vi "SubVI_Stepper_SMC100.vi"(0 "Function":enum16{"Initialize", "Position", "Close"}(ring), 1 "Offset QWP":dbl, 2 "New target position (units)":dbl format="%.2f", 3 "error in (no error)":errorcluster, 4 "Nom de ressource VISA":refnum<visa-resource-name>) -> (5 "Position":dbl, 6 "error out":errorcluster)   [LabVIEW 2025]
panel:
  in  "Timeout (ms)":u32=300
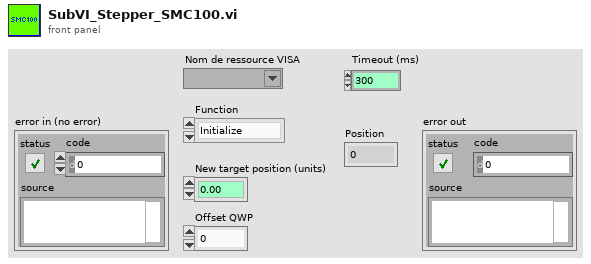
[diagram p1: front panel]
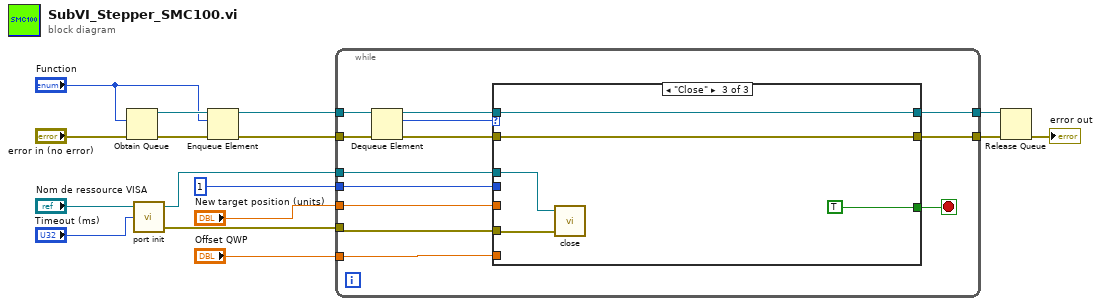
[diagram p0: block diagram]
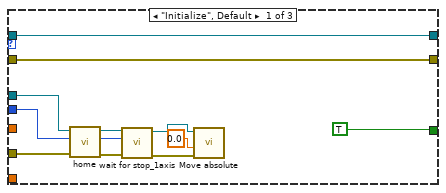
[diagram p2: hidden frame]
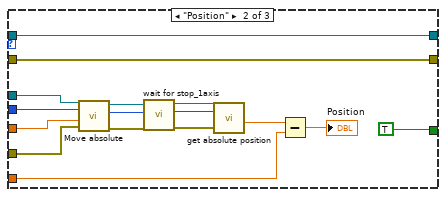
[diagram p3: hidden frame]
diagram:
  n1 = Obtain Queue(element data type="Function", error in (no error)="error in (no error)") -> (queue out=w15:refnum<queue>, error out=w16:errorcluster)  [unwired: 3 in, 1 out]
  n2 = call "port init.vi"("Timeout (ms)"="Timeout (ms)", "Nom de ressource VISA"="Nom de ressource VISA") -> ("error out"=w2:errorcluster, "Visa Handle"=w3:refnum<visa-resource-name>)  [unwired: 2 in]
  n3 = Enqueue Element(queue=w15, element="Function", error in (no error)=w16) -> (queue out=w13:refnum<queue>, error out=w12:errorcluster)  [unwired: 1 in, 1 out]
  n4 = while {
    tunnel: w13 -> [w29]
    tunnel: w12 -> [w28]
    tunnel: [w25] -> w11
    tunnel: [w23] -> w10
    tunnel: w3 -> [w21]
    tunnel: w2 -> [w20]
    tunnel: 1 ("Axis in") -> [w19]
    tunnel: "New target position (units)" -> [w18]
    tunnel: "Offset QWP" -> [w17]
    stop <- w22 stop-if-true
    n5 = Dequeue Element(queue=w29, error in (no error)=w28) -> (queue out=w24:refnum<queue>, element=w27:enum16{"Initialize", "Position", "Close"}, error out=w26:errorcluster)  [unwired: 1 in, 1 out]
    n6 = case shown="\"Close\"" w27 {
      tunnel: w26 -> [w40 w57 w61]
      tunnel: [w40 w57 w61] -> w25
      tunnel: w24 -> [w41 w56 w62]
      tunnel: [w41 w56 w62] -> w23
      tunnel: [TRUE TRUE TRUE] -> w22
      tunnel: w21 -> [w38 w46 w59]
      tunnel: w20 -> [w37 w44 w58]
      tunnel: w19 -> [w36 w45 _]
      tunnel: w18 -> [_ w43 _]
      tunnel: w17 -> [_ w42 _]
      frame "Initialize", Default {
        n7 = call <vilib>:"home.vi"("error in"=w37, "Axis in"=w36, "VISA Handle in"=w38) -> ("error out"=w33:errorcluster, "Axis out"=w34:i32, "VISA Handle out"=w35:refnum<visa-resource-name>)  [unwired: 3 in, 1 out]
        n8 = call "wait for stop_1axis.vi"("error in"=w33, "Axis in"=w34, "VISA Handle in"=w35) -> ("error out"=w31:errorcluster, "VISA Handle out"=w30:refnum<visa-resource-name>)  [unwired: 3 in, 2 out]
        n9 = call "Move absolute.vi"("error in"=w31, "New target position (units)"=0.0, "VISA Handle in"=w30) -> ()  [unwired: 3 in, 4 out]
      }
      frame "Position" {
        n10 = call "Move absolute.vi"("error in"=w44, "New target position (units)"=w43, "Axis in"=w45, "VISA Handle in"=w46) -> ("error out"=w53:errorcluster, "Axis out"=w50:i32, "VISA Handle out"=w54:refnum<visa-resource-name>)  [unwired: 2 in, 1 out]
        n11 = call "wait for stop_1axis.vi"("error in"=w53, "Axis in"=w50, "VISA Handle in"=w54) -> ("error out"=w51:errorcluster, "Axis out"=w49:i32, "VISA Handle out"=w52:refnum<visa-resource-name>)  [unwired: 3 in, 1 out]
        n12 = call "get absolute position.vi"("error in"=w51, "Axis in"=w49, "VISA Handle in"=w52) -> ("Target position (units)"=w48:dbl)  [unwired: 2 in, 4 out]
        n13 = Subtract(x=w48, y=w42) -> (x-y=→"Position":dbl)
      }
      frame "Close" {
        n14 = call "close.vi"("error in"=w58, "VISA Handle in"=w59) -> ()  [unwired: 3 in, 1 out]
      }
    }
  }
  n15 = Release Queue(queue=w10, error in (no error)=w11) -> (error out=→"error out":errorcluster)  [unwired: 1 in, 2 out]
